vi "Cell Photo.vi"(10 "Serial Number":string="1234", 11 "Part Number":string="B0CG1KL3RC") -> (0 "error out":errorcluster, 2 "File ID":string, 3 "Image Path":string)   [LabVIEW 2021]
uses:
  <vilib>/Skyline/File/HTTP/Send File HTTP.vi
  <vilib>/Skyline/File/HTTP/NI Skyline File HTTP.lvclass
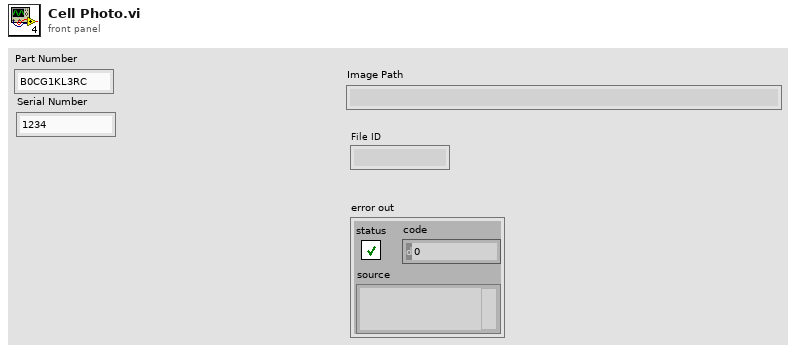
[diagram p1: front panel]
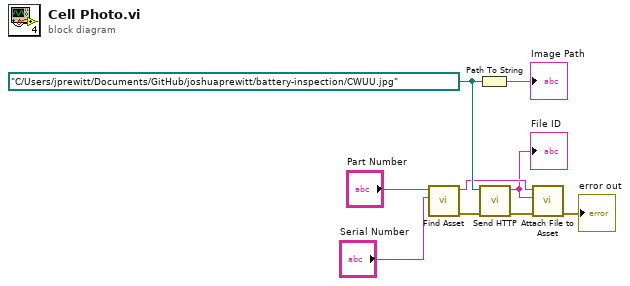
[diagram p0: block diagram]
diagram:
  w6 = path "C:/Users/jprewitt/Documents/GitHub/joshuaprewitt/battery-inspection/CWUU.jpg" ("Path")
  n1 = call "Find Asset.vi"("Serial Number"="Serial Number", "Part Number"="Part Number") -> ("error out"=w4:errorcluster, "Asset ID"=w5:string)  [unwired: 8 in]
  n2 = Path To String(path=w6) -> (string=→"Image Path":string)
  n3 = call-poly <vilib>:"Send HTTP.vi"("error in (no error)"=w4, "path"=w6) -> ("error out"=w3:errorcluster, "id"=w2:string)  [unwired: 7 in]
  "File ID" <- w2
  n4 = call "Attach File to Asset.vi"("error in (no error)"=w3, "File ID"=w2, "Asset ID"=w5) -> ("error out"=→"error out":errorcluster)  [unwired: 8 in]
